vi "File Range.vi"(8 "error in (no error)":errorcluster, 9 "End(%)":dbl, 10 "start(%)":dbl, 11 "Data Load Interface in":refnum<class "Data Load Interface.lvclass">) -> (0 "error out":errorcluster, 3 "Data Load Interface out":refnum<class "Data Load Interface.lvclass">)   [LabVIEW 2020, in "Data Load Interface.lvclass"]
uses:
  Data Load Interface.lvclass
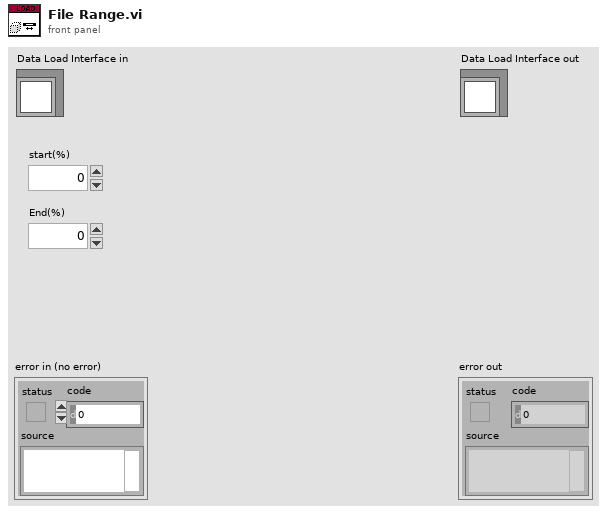
[diagram p1: front panel]
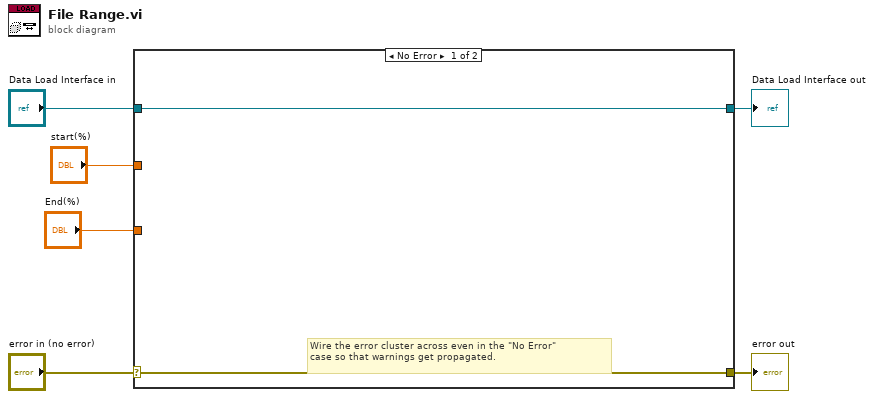
[diagram p0: block diagram]
diagram:
  n1 = case shown="No Error" "error in (no error)" {
    selector: "error in (no error)" -> [w7 w10]
    tunnel: [w7 w10] -> w5
    tunnel: [w8 w9] -> w3
    tunnel: "Data Load Interface in" -> [w8 w9]
    tunnel: "start(%)" -> [_ _]
    tunnel: "End(%)" -> [_ _]
    frame No Error {
      # "Wire the error cluster across even in the \"No Error\"\ncase so that warnings get propagated."
    }
    frame Error {
    }
  }
  "error out" <- w5
  "Data Load Interface out" <- w3
